vi "Model Update Duration.vi"(8 "error in (no error)":errorcluster, 10 "Duration":dbl, 11 "Chef Model in":refnum<class "Chef Model.lvclass">) -> (0 "error out":errorcluster, 3 "Chef Model out":refnum<class "Chef Model.lvclass">)   [LabVIEW 2024, in "Chef Model.lvlib" / "Chef Model.lvclass"]
uses:
  Chef Model.lvclass
  Chef Model.lvclass/Chef Model.ctl
  Chef Controller/Chef Controller Messages/Controller Update Duration Msg/Controller Update Duration Msg.lvclass/Controller Update Duration Msg.ctl
  <vilib>/ActorFramework/Message Enqueuer/Message Enqueuer.lvclass/Message Enqueuer.ctl
  <vilib>/ActorFramework/Message Enqueuer/Enqueue.vi
  Chef Controller/Chef Controller Messages/Controller Update Duration Msg/Controller Update Duration Msg.lvclass
  C:/Program Files/National Instruments/LabVIEW 2024/vi.lib/ActorFramework/Message/Message.lvclass
  <vilib>/ActorFramework/Message Priority Queue/Priority Enqueue.vi
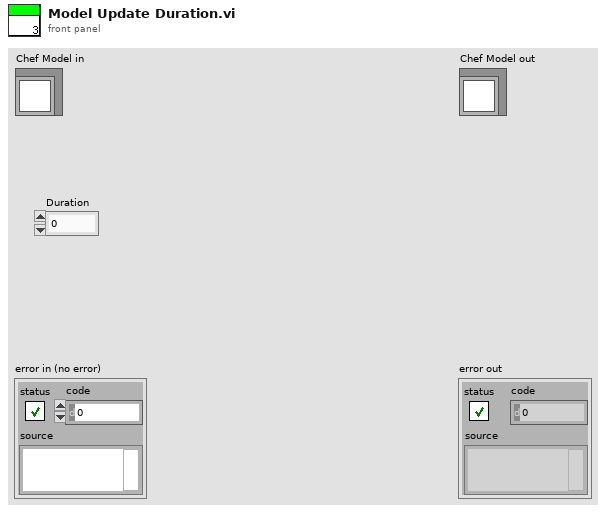
[diagram p1: front panel]
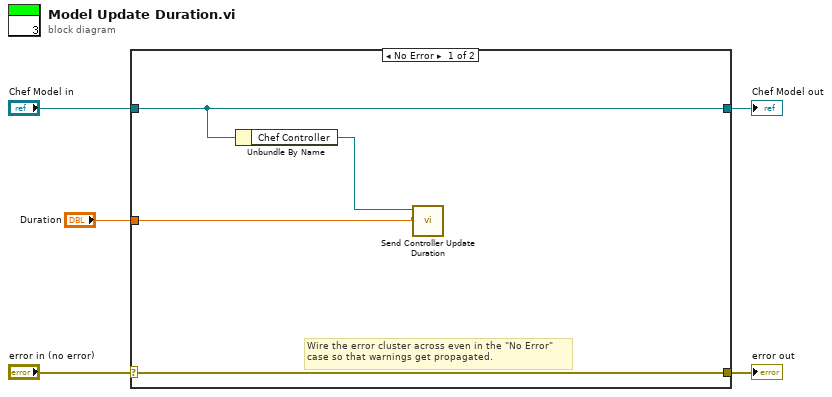
[diagram p0: block diagram]
diagram:
  n1 = case shown="No Error" "error in (no error)" {
    selector: "error in (no error)" -> [w9 w11]
    tunnel: [w9 w11] -> w4
    tunnel: [w8 w10] -> w2
    tunnel: "Chef Model in" -> [w8 w10]
    tunnel: "Duration" -> [w6 _]
    frame No Error {
      # "Wire the error cluster across even in the \"No Error\"\ncase so that warnings get propagated."
      n2 = Unbundle By Name(w8) -> ("Chef Controller"=w7:refnum<class "Message Enqueuer.lvclass">)
      n3 = call "Send Controller Update Duration.vi"("Duration"=w6, "Message Enqueuer"=w7) -> ()  [unwired: 8 in, 2 out]
    }
    frame Error {
    }
  }
  "error out" <- w4
  "Chef Model out" <- w2
